vi "Serial write template.vi"   [LabVIEW 2020]
uses:
  <vilib>/Aledyne-TSXperts/Arduino Compatible Compiler for LabVIEW/Code Generator/Arduino APIs/Serial/Serial Settings.ctl
  <vilib>/Aledyne-TSXperts/Arduino Compatible Compiler for LabVIEW/Code Generator/Arduino APIs/Digital/PinDirection.ctl
  <vilib>/Aledyne-TSXperts/Arduino Compatible Compiler for LabVIEW/Arduino Compatible Compiler for LabVIEW.lvlib
types:
  T1 = typedef "Arduino Compatible Compiler for LabVIEW.lvlib/PinDirection.ctl" = enum16{" INPUT", "OUTPUT", " INPUT_PULLUP"}
  T2 = typedef "Arduino Compatible Compiler for LabVIEW.lvlib/Serial Settings.ctl" = u16
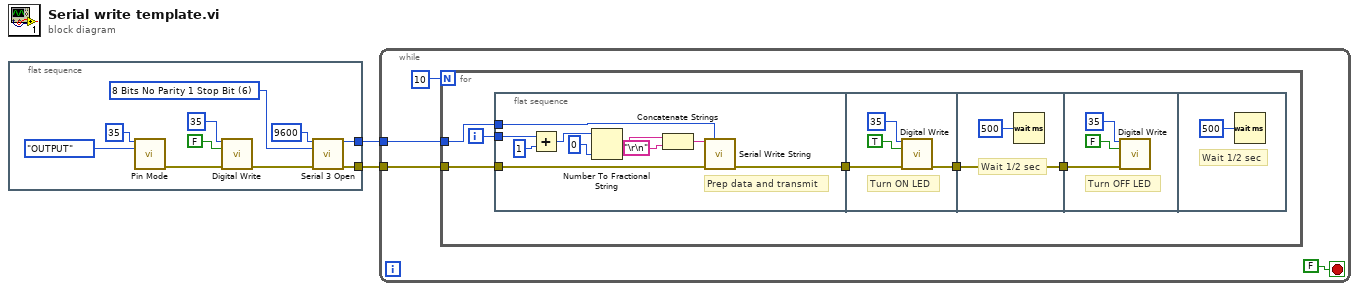
[diagram p0: block diagram]
diagram:
  n1 = flat-sequence {
    tunnel: [w12] -> w2
    tunnel: [w11] -> w1
    frame #0 {
      w9 = T2 6 items=["5 Bits No Parity 1 Stop Bit"=0, "6 Bits No Parity 1 Stop Bit"=2, "7 Bits No Parity 1 Stop Bit"=4, "8 Bits No Parity 1 Stop Bit"=6, "5 Bits No Parity 2 Stop Bits"=8, "6 Bits No Parity 2 Stop Bits"=10, "7 Bits No Parity 2 Stop Bits"=12, "8 Bits No Parity 2 Stop Bits"=14, "5 Bits Even Parity 1 Stop Bits"=32, "6 Bits Even Parity 1 Stop Bits"=34, "7 Bits Even Parity 1 Stop Bits"=36, "8 Bits Even Parity 1 Stop Bits"=38, "5 Bits Even Parity 2 Stop Bits"=40, "6 Bits Even Parity 2 Stop Bits"=42, "7 Bits Even Parity 2 Stop Bits"=44, "8 Bits Even Parity 2 Stop Bits"=46, "5 Bits Odd Parity 1 Stop Bits"=48, "6 Bits Odd Parity 1 Stop Bits"=50, "7 Bits Odd Parity 1 Stop Bits"=52, "8 Bits Odd Parity 1 Stop Bits"=54, "5 Bits Odd Parity 2 Stop Bits"=56, "6 Bits Odd Parity 2 Stop Bits"=58, "7 Bits Odd Parity 2 Stop Bits"=60, "8 Bits Odd Parity 2 Stop Bits"=62] ("Serial Settings")
      n2 = call <vilib>:"Pin Mode.vi"("pin"=u8 35, "direction"=PinDirection."OUTPUT") -> ("error out"=w4:errorcluster)  [unwired: 13 in]
      n3 = call <vilib>:"Digital Write.vi"("pin"=u8 35, "state"=FALSE, "error in (no error)"=w4) -> ("error out"=w3:errorcluster)  [unwired: 12 in]
      n4 = call <vilib>:"Serial 3 Open.vi"("Speed"=u32 9600, "Serial Settings"=w9, "error in (no error)"=w3) -> ("Instance"=w11:u8, "error out"=w12:errorcluster)  [unwired: 11 in]
    }
  }
  n5 = while {
    tunnel: w2 -> [w14]
    tunnel: w1 -> [w15]
    stop <- FALSE stop-if-true
    n6 = for {
      N: 10 -> [_]
      tunnel: w15 -> [w22]
      tunnel: w14 -> [w21]
      i -> [w20]
      n7 = flat-sequence {
        tunnel: w20 -> [w24]
        tunnel: w22 -> [w31]
        tunnel: w21 -> [w30]
        tunnel: [w26] -> w19
        tunnel: w19 -> [w36]
        tunnel: [w33] -> w17
        tunnel: [w37] -> w18
        tunnel: w17 -> [w37]
        tunnel: w18 -> [w39]
        frame #0 {
          # "Prep data and transmit"
          n8 = Add(x=w24, y=1) -> (x+y=w23:i32)
          n9 = Number To Fractional String(number=w23, precision (6)=i16 0) -> (F-format string=w28:string)  [unwired: 2 in]
          n10 = Concatenate Strings(w28, "\r\n") -> (w27:string)
          n11 = call <vilib>:"Serial Write String.vi"("String"=w27, "Instance"=w31, "error in (no error)"=w30) -> ("error out"=w26:errorcluster)  [unwired: 12 in]
        }
        frame #1 {
          # "Turn ON LED"
          n12 = call <vilib>:"Digital Write.vi"("pin"=u8 35, "state"=TRUE, "error in (no error)"=w36) -> ("error out"=w33:errorcluster)  [unwired: 12 in]
        }
        frame #2 {
          # "Wait 1/2 sec"
          n13 = Wait (ms)(milliseconds to wait=u32 500) -> ()  [unwired: 1 out]
        }
        frame #3 {
          # "Turn OFF LED"
          n14 = call <vilib>:"Digital Write.vi"("pin"=u8 35, "state"=FALSE, "error in (no error)"=w39) -> ()  [unwired: 12 in, 1 out]
        }
        frame #4 {
          # "Wait 1/2 sec"
          n15 = Wait (ms)(milliseconds to wait=u32 500) -> ()  [unwired: 1 out]
        }
      }
    }
  }
